vi "Lesson8 - multiple while loops Local Variable STOP.vi"() -> ()   [LabVIEW 2013]
panel:
  in  "Stop Button":bool
  out "Numeric 4":i32
  out "Numeric 3":i32
  in  "stop":bool
  out "Numeric 2":i32
  out "Numeric":i32
  # "cannot use latch action when using local variables.\n\nso, can choose switch when released"
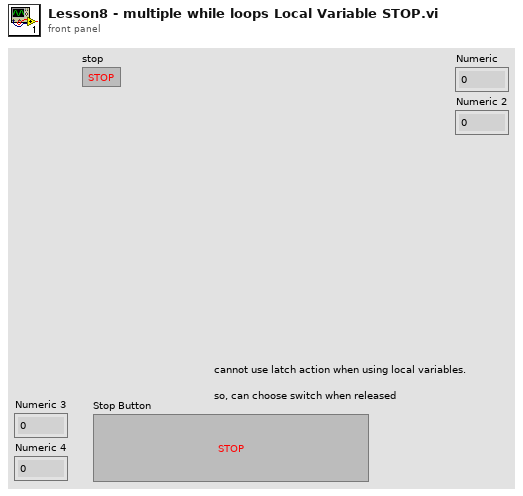
[diagram p1: front panel]
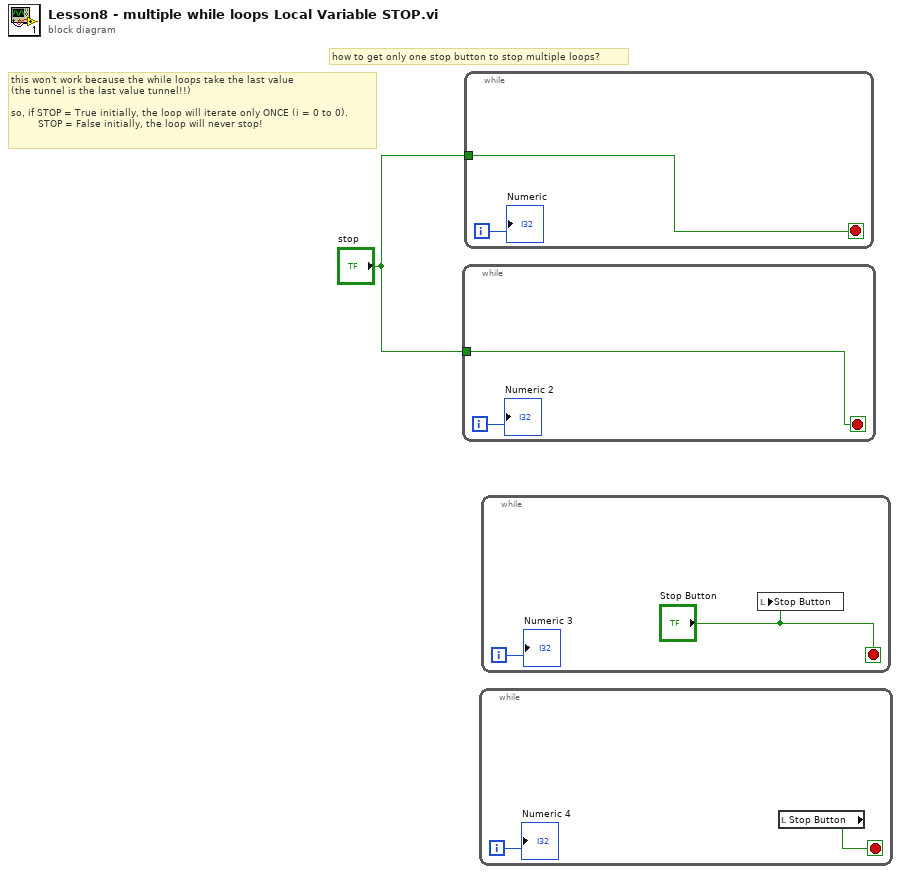
[diagram p0: block diagram]
diagram:
  # "this won't work because the while loops take the last value \n(the tunnel is the last value tunnel!!)\n\nso, if STOP = True initially, the loop will iterate only ONCE (i = 0 to 0).\n         STOP = False initially, the loop will never stop!"
  # "how to get only one stop button to stop multiple loops?"
  n1 = while {
    tunnel: "stop" -> [w2]
    i -> [w3]
    stop <- w2 stop-if-true
    "Numeric 2" <- w3
  }
  n2 = while {
    tunnel: "stop" -> [w4]
    i -> [w5]
    stop <- w4 stop-if-true
    "Numeric" <- w5
  }
  n3 = while {
    i -> [w7]
    stop <- w6 stop-if-true
    n4 = local read "Stop Button"() -> (w6:bool)
    "Numeric 4" <- w7
  }
  n5 = while {
    i -> [w9]
    stop <- "Stop Button" stop-if-true
    n6 = local write "Stop Button"("Stop Button") -> ()
    "Numeric 3" <- w9
  }
